vi "Usuwanie punktu z listy współrzędnych.vi"(10 "Lista współrzędnych":string[][](array[string]), 11 "Lista z punktami do usunięcia":refnum<vi>) -> (3 "Lista współrzędnych 2":string[][](array[string]))   [LabVIEW 2015, in "Biblioteka moduł map v3.lvlib" / "Obsługa listy współrzędnych.lvlib"]
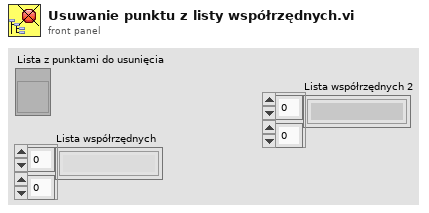
[diagram p1: front panel]
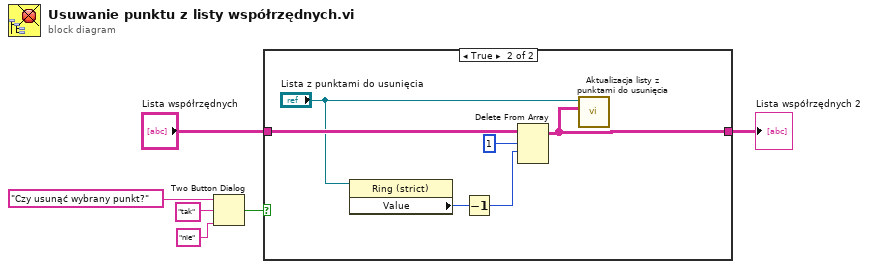
[diagram p0: block diagram]
diagram:
  n1 = Two Button Dialog(message="Czy usunąć wybrany punkt?", 1:"nie" ("F button name (\"Cancel\")"), 2:"tak" ("T button name (\"OK\")")) -> (T button?=w2:bool)
  n2 = case shown="True" w2 {
    tunnel: "Lista współrzędnych" -> [w7 w11]
    tunnel: [w7 w10] -> w1
    frame False {
    }
    frame True {
      n3 = property class="Ring (strict)"(reference="Lista z punktami do usunięcia") -> ("Value"=w8:u16)  [unwired: 1 in, 2 out]
      n4 = Decrement(x=w8) -> (x-1=w12:u16)
      n5 = Delete From Array(array=w11, length=1, index (row)=w12) -> (array with subset deleted=w10:string[][])  [unwired: 1 in, 1 out]
      n6 = call "Aktualizacja listy z punktami do usunięcia.vi"("Lista współrzędnych"=w10, "Lista z punktami do usunięcia"="Lista z punktami do usunięcia") -> ()  [unwired: 10 in]
    }
  }
  "Lista współrzędnych 2" <- w1
